vi "Latihan.vi"() -> ()   [LabVIEW 2015]
uses:
  sub latihan/Control 4.ctl
panel:
  in  "Lower Limit":dbl
  in  "Upper Limit":dbl
  in  "Stop Button":bool
  out "Warning":string
  out "Temperature History":dbl(graph)
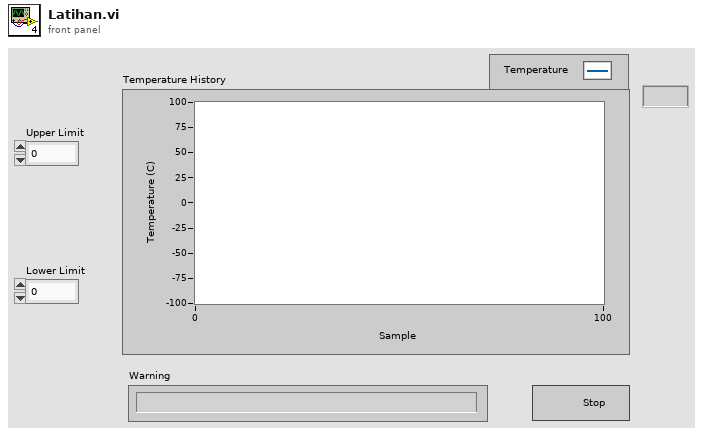
[diagram p1: front panel]
types:
  T1 = typedef "Control 4.ctl" = cluster{"Current Temperature":dbl, "Max Temperature":dbl, "Min Temperature 2":dbl, "Temperature Warning?":bool, "Termperature Warning Text":string}
  T2 = enum16{"Acquisition", "Range Check", "Analysis", "Data Log", "Time Check"}
  T3 = enum16{"open", "replace", "create", "open or create", "replace or create", "replace or create with confirmation"}
  T4 = cluster{"Current Temperaturel":dbl, "Max Temperature":dbl, "Min Temperature":dbl, "Temperature Warning":bool, "Temperature Warning Text":string}
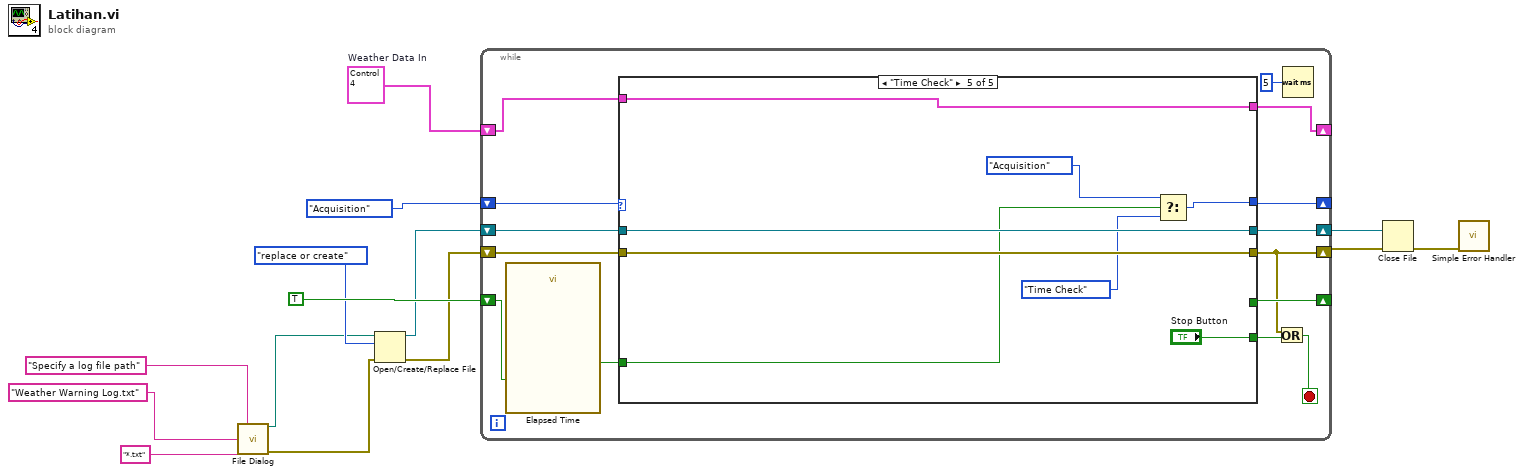
[diagram p0: block diagram]
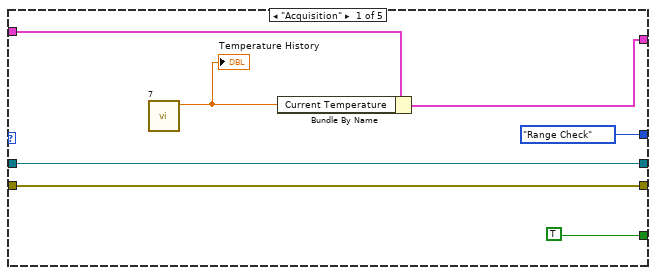
[diagram p2: hidden frame]
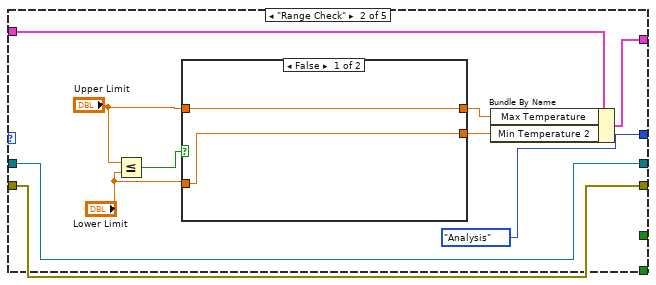
[diagram p3: hidden frame]
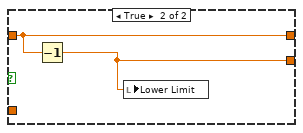
[diagram p4: hidden frame]
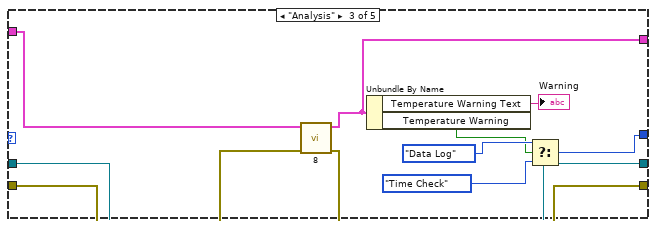
[diagram p5: hidden frame]
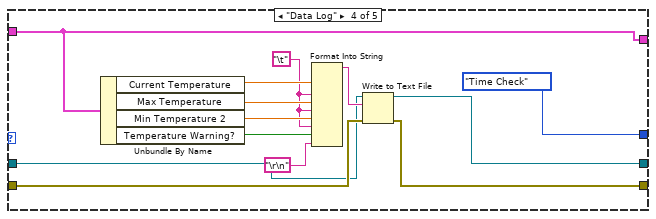
[diagram p6: hidden frame]
diagram:
  w1 = T1 {"Current Temperature"=0.0, "Max Temperature"=0.0, "Min Temperature 2"=0.0, "Temperature Warning?"=FALSE, "Termperature Warning Text"="No Warning"}  # Weather Data In
  n1 = call "File Dialog"("prompt"="Specify a log file path", "default name"="Weather Warning Log.txt", "pattern (all files)"="*.txt" ("pattern label")) -> ("selected path"=w6:path, "error out"=w10:errorcluster)  [unwired: 9 in, 2 out]
  n2 = Open/Create/Replace File(file path (use dialog)=w6, error in=w10, operation (0:open)=T3."replace or create") -> (refnum out=w5:refnum<file>, error out=w12:errorcluster)  [unwired: 3 in, 1 out]
  n3 = while {
    shift-right: [w22] -> _
    shift-left: TRUE -> [w18]
    shift-right: [w21] -> w11
    shift-left: w12 -> [w27]
    shift-right: [w23] -> w4
    shift-left: w5 -> [w24]
    shift-right: [w19] -> _
    shift-left: T2."Acquisition" -> [w20]
    shift-right: [w15] -> _
    shift-left: w1 -> [w16]
    stop <- w25 stop-if-true
    n4 = call "Elapsed Time"("Reset"=w18) -> ("Time has Elapsed"=w26:bool)  [unwired: 11 in, 7 out]
    n5 = case shown="\"Time Check\"" w20 {
      tunnel: w27 -> [w34 w39 w57 w64 w80]
      tunnel: [w34 w39 w56 w63 w80] -> w21
      tunnel: w26 -> [_ _ _ _ w78]
      tunnel: w24 -> [w33 w40 w58 w62 w79]
      tunnel: [w33 w40 w58 w61 w79] -> w23
      tunnel: [TRUE ("stop") _ _ _ _] -> w22
      tunnel: [T2."Range Check" T2."Analysis" w53 T2."Time Check" w75] -> w19
      tunnel: [_ _ _ _ "Stop Button"] -> w17
      tunnel: w16 -> [w30 w37 w51 w60 w73]
      tunnel: [w29 w36 w50 w60 w73] -> w15
      frame "Acquisition" {
        n6 = call "7.vi"() -> ("Temperature Value"=w35:dbl)  [unwired: 11 in]
        "Temperature History" <- w35
        n7 = Bundle By Name(cluster=w30, "Current Temperature"=w35) -> (w29:T1)
      }
      frame "Range Check" {
        n8 = Less Or Equal?(x="Upper Limit", y="Lower Limit") -> (x <= y?=w43:bool)
        n9 = case shown="False" w43 {
          tunnel: "Upper Limit" -> [w47 w48]
          tunnel: "Lower Limit" -> [w46 _]
          tunnel: [w46 w49] -> w42
          tunnel: [w47 w48] -> w41
          frame False {
          }
          frame True {
            n10 = Decrement(x=w48) -> (x-1=w49:dbl)
            n11 = local write "Lower Limit"(w49) -> ()
          }
        }
        n12 = Bundle By Name(cluster=w37, "Max Temperature"=w41, "Min Temperature 2"=w42) -> (w36:T1)
      }
      frame "Analysis" {
        n13 = call "8.vi"("error in (no error)"=w57, "Weather Data In"=w51) -> ("error out"=w56:errorcluster, "Weather Data Out"=w50:T4)  [unwired: 8 in]
        n14 = Unbundle By Name(w50) -> ("Temperature Warning Text"=→"Warning":string, "Temperature Warning"=w52:bool)
        n15 = Select(t=T2."Data Log", s=w52, f=T2."Time Check") -> (s? t:f=w53:T2)
      }
      frame "Data Log" {
        w67 = "\t"
        n16 = Unbundle By Name(w60) -> ("Current Temperature"=w68:dbl, "Max Temperature"=w69:dbl, "Min Temperature 2"=w70:dbl, "Temperature Warning?"=w71:bool)
        n17 = Format Into String(w68, w67, w69, w67, w70, w67, w71, "\r\n") -> (resulting string=w66:string)  [unwired: 3 in, 1 out]
        n18 = Write to Text File(file (use dialog)=w62, text=w66, error in=w64) -> (refnum out=w61:refnum<file>, error out=w63:errorcluster)  [unwired: 1 in, 1 out]
      }
      frame "Time Check" {
        n19 = Select(t=T2."Acquisition", s=w78, f=T2."Time Check") -> (s? t:f=w75:T2)
      }
    }
    n20 = Or(x=w21, y=w17) -> (x .or. y?=w25:bool)
    n21 = Wait (ms)(milliseconds to wait=u32 5 ("y")) -> ()  [unwired: 1 out]
  }
  n22 = Close File(refnum=w4, error in=w11) -> (error out=w3:errorcluster)  [unwired: 1 out]
  n23 = call <vilib>:"Simple Error Handler.vi"("error in (no error)"=w3) -> ()  [unwired: 4 in, 5 out]
